vi "DB Create Tables.vi"(8 "error in (no error)":errorcluster, 9 "Create Table":T3={"table"="", "column information"=[], "primary key (-1)"=-1, "use file? (F)"=FALSE}, 11 "MYSQL Database in":refnum<class "MYSQL Database.lvclass">) -> (0 "error out":errorcluster, 3 "MYSQL Database out":refnum<class "MYSQL Database.lvclass">)   [LabVIEW 2023, in "HardwareAbstractionLayer_LVOOP.lvlib" / "MYSQL Database.lvclass"]
uses:
  MYSQL Database.lvclass
  <vilib>/addons/database/Auxilliary.llb/DB Tools Column Info.ctl
  <vilib>/addons/database/Auxilliary.llb/DB Tools DataTypes.ctl
  MYSQL Database.lvclass/MYSQL Database.ctl
  <vilib>/addons/database/NI_Database_API.lvlib
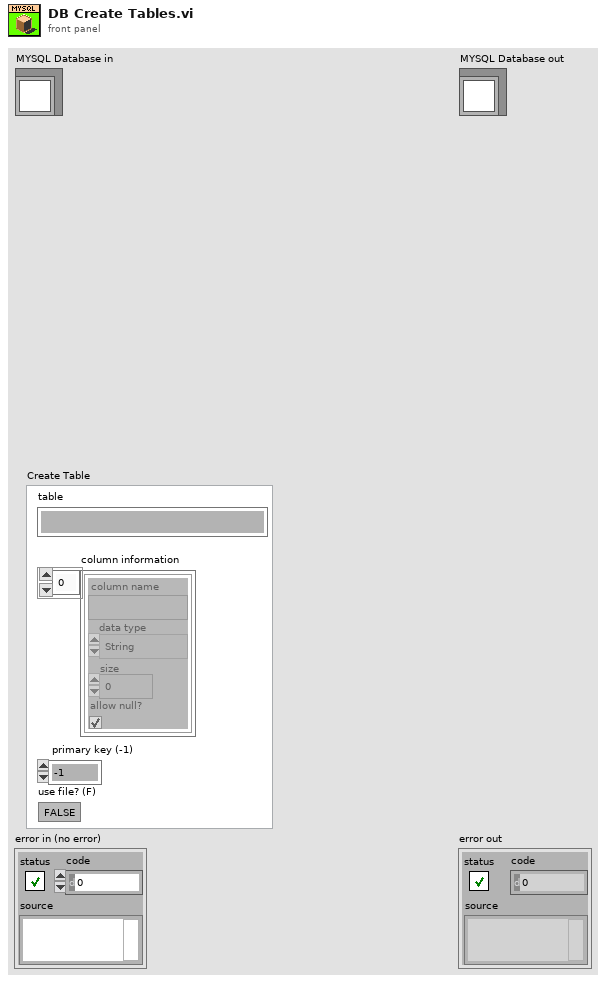
[diagram p1: front panel]
types:
  T1 = typedef "NI_Database_API.lvlib/DB Tools Column Info.ctl" = cluster{"column name":string, "data type":T2, "size":i32, "allow null?":bool}
  T2 = typedef "NI_Database_API.lvlib/DB Tools DataTypes.ctl" = enum16{"String", "Long (I32)", "Single (SGL)", "Double (DBL)", "Date/Time", "Binary"}
  T3 = cluster{"table":string, "column information":T1[], "primary key (-1)":i32, "use file? (F)":bool}
  T4 = typedef "NI_Database_API.lvlib/Conn ObjectReference.ctl" = refnum<k1>
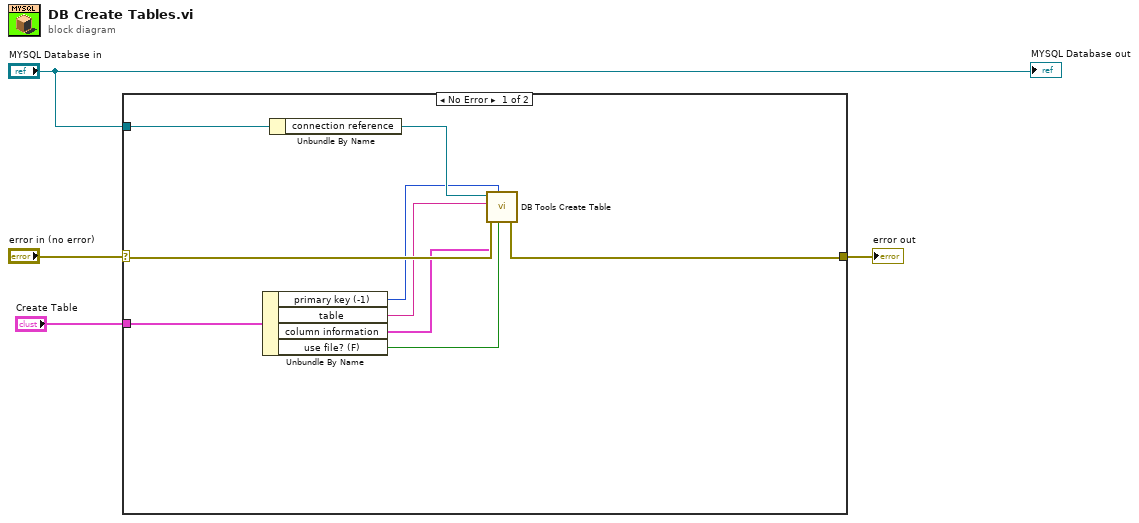
[diagram p0: block diagram]
diagram:
  n1 = case shown="No Error" "error in (no error)" {
    selector: "error in (no error)" -> [w11 w14]
    tunnel: "MYSQL Database in" -> [w13 _]
    tunnel: [w12 w14] -> w2
    tunnel: "Create Table" -> [w9 _]
    frame No Error {
      n2 = Unbundle By Name(w9) -> ("primary key (-1)"=w5:i32, "table"=w8:string, "column information"=w7:T1[], "use file? (F)"=w6:bool)
      n3 = Unbundle By Name(w13) -> ("connection reference"=w10:T4)
      n4 = call <vilib>:"DB Tools Create Table.vi"("use file? (F)"=w6, "primary key (-1)"=w5, "error in (no error)"=w11, "column information"=w7, "table"=w8, "connection reference"=w10) -> ("error out"=w12:errorcluster)  [unwired: 2 in, 1 out]
    }
    frame Error {
    }
  }
  "error out" <- w2
  "MYSQL Database out" <- "MYSQL Database in"
